vi "Limit Accel Indices.vi"(7 "Last Accel":bool, 9 "Size":i32, 10 "Decel":i32[](array[numeric]), 11 "Accel":i32[](array[numeric])) -> (2 "Decel Index":i32, 3 "Accel Index":i32)   [LabVIEW 2018]
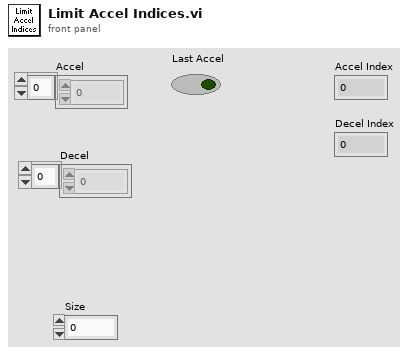
[diagram p1: front panel]
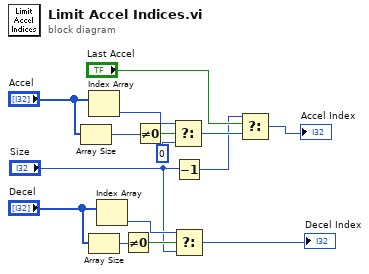
[diagram p0: block diagram]
diagram:
  n1 = Array Size(array="Accel") -> (size(s)=w3:i32)
  n2 = Index Array(array="Accel") -> (element=w14:i32)  [unwired: 1 in]
  n3 = Array Size(array="Decel") -> (size(s)=w11:i32)
  n4 = Index Array(array="Decel") -> (element=w12:i32)  [unwired: 1 in]
  n5 = Not Equal To 0?(x=w11) -> (x != 0?=w10:bool)
  n6 = Not Equal To 0?(x=w3) -> (x != 0?=w15:bool)
  n7 = Select(t=w14, s=w15, f=0) -> (s? t:f=w6:i32)
  n8 = Decrement(x="Size") -> (x-1=w2:i32)
  n9 = Select(t=w12, s=w10, f="Size") -> (s? t:f=→"Decel Index":i32)
  n10 = Select(t=w2, s="Last Accel", f=w6) -> (s? t:f=→"Accel Index":i32)
